vi "Get Pressure Servo Valve Value.vi"(8 "error in (no error)":errorcluster, 11 "ILC PSV Open Loop Actuator Cylinder in":refnum<class "ILC PSV Open Loop Actuator Cylinder.lvclass">) -> (0 "error out":errorcluster, 2 "Value":dbl format="%.2f", 3 "ILC PSV Open Loop Actuator Cylinder out":refnum<class "ILC PSV Open Loop Actuator Cylinder.lvclass">)   [LabVIEW 2015, in "ILC PSV Open Loop Actuator Cylinder.lvclass"]
uses:
  ILC PSV Open Loop Actuator Cylinder.lvclass
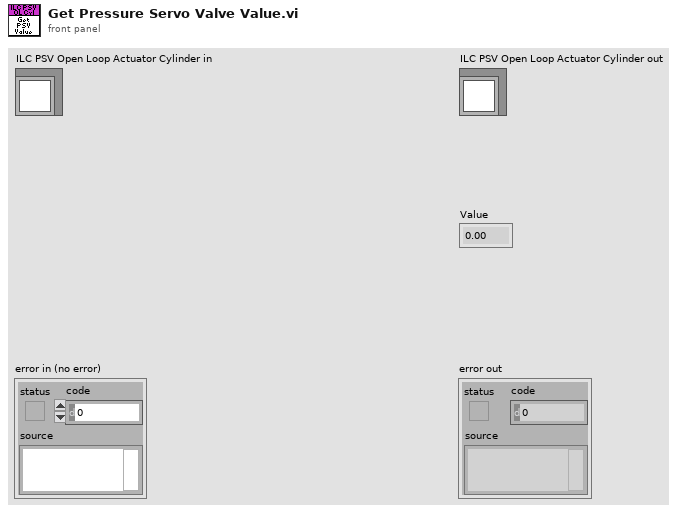
[diagram p1: front panel]
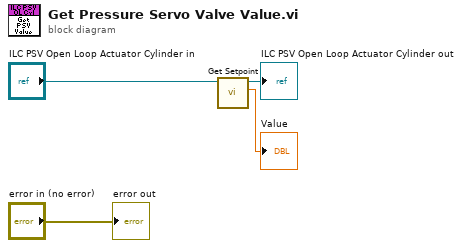
[diagram p0: block diagram]
diagram:
  n1 = call-dynamic "Get Setpoint.vi"("ILC Actuator Cylinder in"="ILC PSV Open Loop Actuator Cylinder in") -> ("Setpoint"=→"Value":dbl, "ILC Actuator Cylinder out"=→"ILC PSV Open Loop Actuator Cylinder out":refnum<class "ILC PSV Open Loop Actuator Cylinder.lvclass">)  [unwired: 9 in]
  "error out" <- "error in (no error)"
